vi "sir_v3.vi"() -> ()   [LabVIEW 2009]
panel:
  out "Numarul de caractere":dbl
  in  "stop":bool
  out "Sir de caractere cu majuscule":string="APLICATIE LABWIEW\n"
  in  "Sir de caractere cu majuscule si minuscule":string="Aplicatie LabWIEW\n"
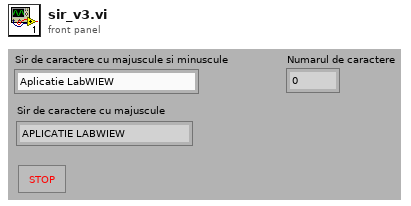
[diagram p1: front panel]
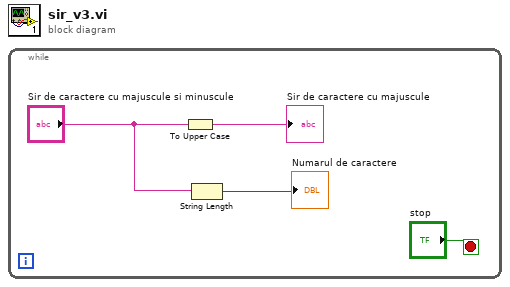
[diagram p0: block diagram]
diagram:
  n1 = while {
    stop <- "stop" stop-if-true
    n2 = To Upper Case(1:"Sir de caractere cu majuscule si minuscule") -> (0:→"Sir de caractere cu majuscule":string)
    n3 = String Length(string="Sir de caractere cu majuscule si minuscule") -> (length=→"Numarul de caractere":i32)
  }
